vi "tcs shm log Event Filter Change In Position LV.vi"(8 "error in (no error)":errorcluster, 11 "logevent_FilterChangeInPosition_Ctl":T1) -> (0 "error out":errorcluster, 2 "function return":i32, 3 "logevent_FilterChangeInPosition_Ctl out":T1)   [LabVIEW 2016, in "SALLV_tcs.lvlib"]
doc: "int tcs_shm_logEvent_FilterChangeInPositionLV(tcs_logevent_FilterChangeInPositionLV *logevent_FilterChangeInPosition_Ctl );"
uses:
  SALLV_tcs.lvlib
  SALLV_tcs.so
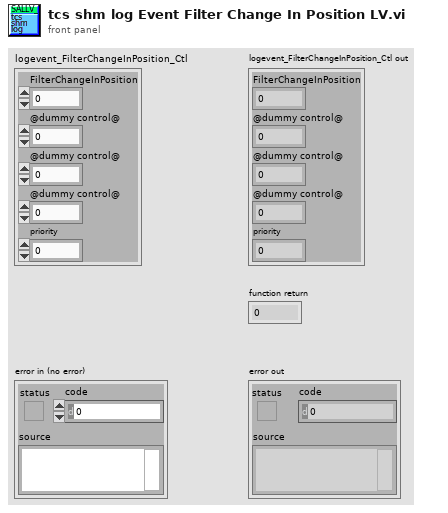
[diagram p1: front panel]
types:
  T1 = cluster{"FilterChangeInPosition":u8, "@dummy control@":i8, "@dummy control@":i8, "@dummy control@":i8, "priority":i32}
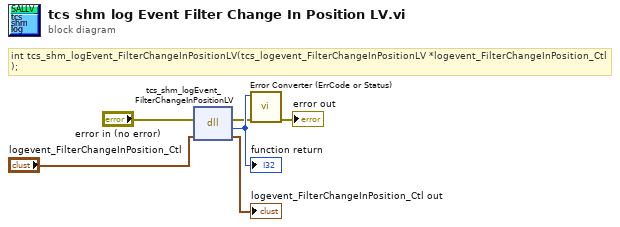
[diagram p0: block diagram]
diagram:
  # "int tcs_shm_logEvent_FilterChangeInPositionLV(tcs_logevent_FilterChangeInPositionLV *logevent_FilterChangeInPosition_Ctl );"
  n1 = dll-call lib="home/andres/Desktop/SALLV_tcs/SALLV_tcs.*" fn="tcs_shm_logEvent_FilterChangeInPositionLV"(error in="error in (no error)", "logevent_FilterChangeInPosition_Ctl"="logevent_FilterChangeInPosition_Ctl") -> (error out=w2:errorcluster, w6:i32, "logevent_FilterChangeInPosition_Ctl"=→"logevent_FilterChangeInPosition_Ctl out":T1)  [unwired: 2 in, 1 out]
  "function return" <- w6
  n2 = call "Error Converter (ErrCode or Status).vi"("error in (no error)"=w2, "error code"=w6) -> ("error out"=→"error out":errorcluster)  [unwired: 9 in]
